vi "DSRead Variant.vi"(6 "wait for updated value (T)":bool, 8 "error in":errorcluster[](array[cluster]), 9 "ms timeout (10000)":i32, 11 "connection in":refnum<k13>[](array[refnum])) -> (0 "error out":errorcluster[](array[cluster]), 2 "data":variant[](array[variant]), 3 "connection out":refnum<k13>[](array[refnum]))   [LabVIEW 2011]
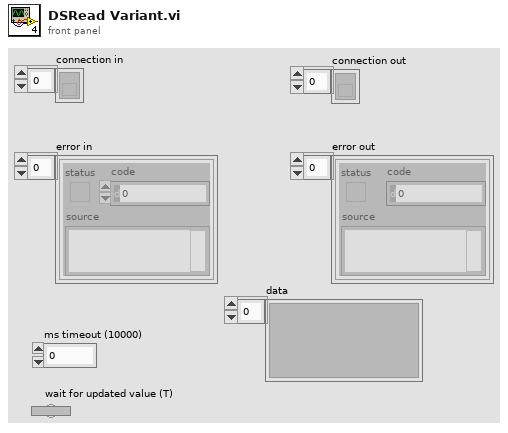
[diagram p1: front panel]
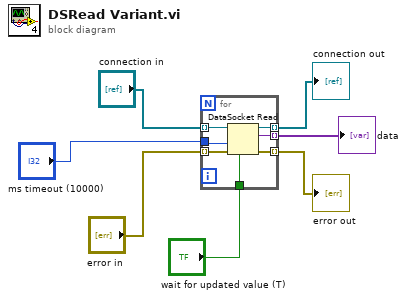
[diagram p0: block diagram]
diagram:
  n1 = for {
    tunnel: [w14] -> w4 mode=indexing
    tunnel: [w13] -> w5 mode=indexing
    tunnel: [w8] -> w1 mode=indexing
    tunnel: "connection in" -> [w12] mode=indexing
    tunnel: "error in" -> [w11] mode=indexing
    tunnel: "ms timeout (10000)" -> [w10]
    tunnel: "wait for updated value (T)" -> [w9]
    n2 = DataSocket Read(6:w9, 8:w11, 9:w10, 11:w12) -> (0:w14:errorcluster, 2:w8:variant, 3:w13:refnum<k13>)  [unwired: 1 in, 4 out]
  }
  "connection out" <- w5
  "error out" <- w4
  "data" <- w1
